vi "MGI-Wait ms.vi"(6 "ms":u32, 7 "Error In":errorcluster) -> (3 "Error Out":errorcluster)   [LabVIEW 2021]
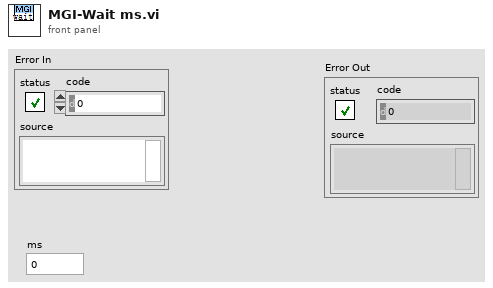
[diagram p1: front panel]
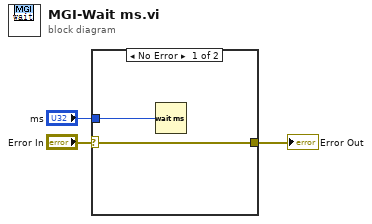
[diagram p0: block diagram]
diagram:
  n1 = case shown="No Error" "Error In" {
    selector: "Error In" -> [w4 w6]
    tunnel: "ms" -> [w5 _]
    tunnel: [w4 w6] -> w3
    frame No Error {
      n2 = Wait (ms)(milliseconds to wait=w5) -> ()  [unwired: 1 out]
    }
    frame Error {
    }
  }
  "Error Out" <- w3
